vi "Save.vi"(8 "error in (no error)":errorcluster, 9 "new command":string, 10 "Msg in":T1, 11 "FakePressureController in":refnum<class "SMC100.lvclass">) -> (0 "error out":errorcluster, 1 "Path":path, 2 "Msg out":T1, 3 "FakePressureController out":refnum<class "SMC100.lvclass">, 4 "new command":string)   [LabVIEW 2020, in "SMC100.lvclass"]
uses:
  SMC100.lvclass
  DriverMsg.ctl
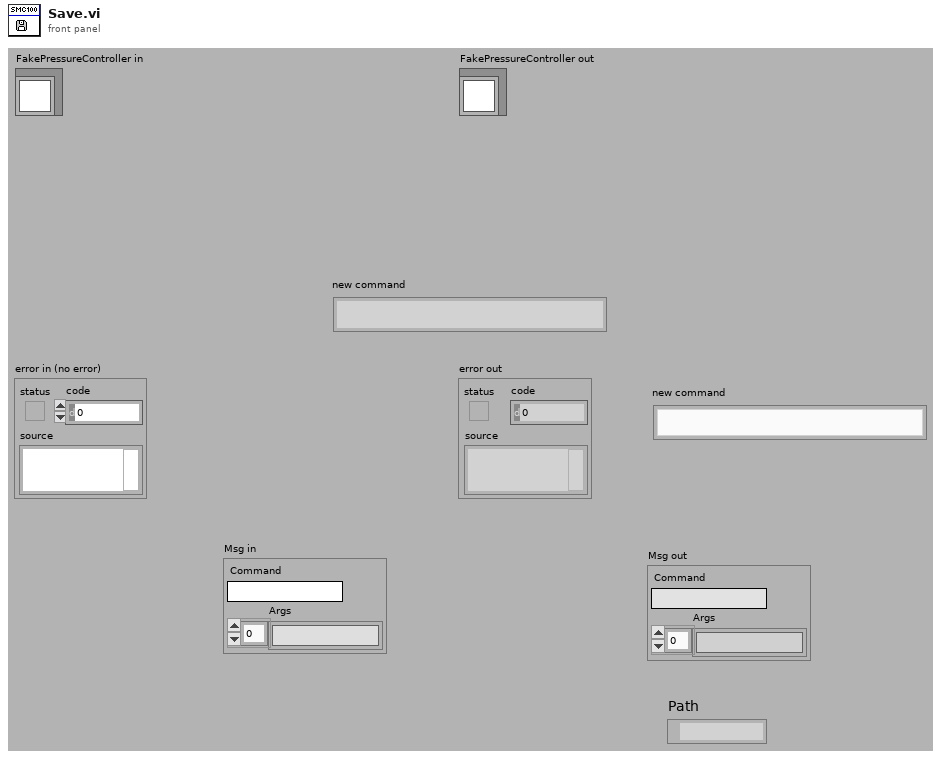
[diagram p1: front panel]
types:
  T1 = typedef "DriverMsg.ctl" = cluster{"Command":string, "Args":string[]}
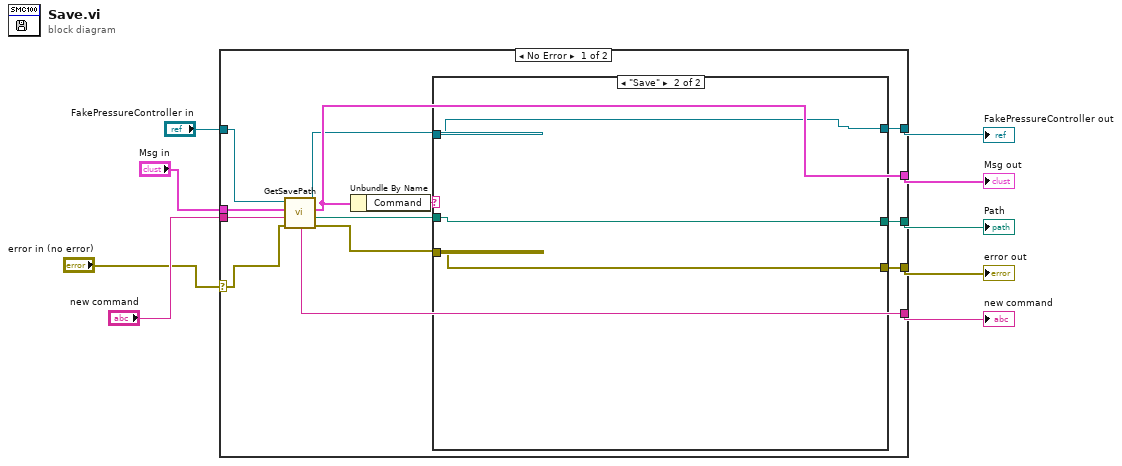
[diagram p0: block diagram]
diagram:
  n1 = case shown="No Error" "error in (no error)" {
    selector: "error in (no error)" -> [w18 w32]
    tunnel: "Msg in" -> [w22 w30]
    tunnel: "new command" -> [w21 w31]
    tunnel: [w20 w31] -> w7
    tunnel: [w12 w32] -> w6
    tunnel: [w10 _] -> w5
    tunnel: [w17 w30] -> w4
    tunnel: "FakePressureController in" -> [w19 w29]
    tunnel: [w14 w29] -> w2
    frame No Error {
      n2 = call-dynamic "GetSavePath.vi"("error in (no error)"=w18, "new command"=w21, "Msg in"=w22, "BaseDriver in"=w19) -> ("error out"=w13:errorcluster, "Path"=w11:path, "Msg out"=w17:T1, "BaseDriver out"=w15:refnum<class "SMC100.lvclass">, "new command"=w20:string)  [unwired: 3 in]
      n3 = Unbundle By Name(w17) -> ("Command"=w16:string)
      n4 = case shown="\"Save\"" w16 {
        tunnel: w15 -> [w25 w28]
        tunnel: [w25 w28] -> w14
        tunnel: w13 -> [w24 w27]
        tunnel: [w24 w27] -> w12
        tunnel: w11 -> [w23 w26]
        tunnel: [w23 w26] -> w10
        frame "False", Default {
        }
        frame "Save" {
        }
      }
    }
    frame Error {
    }
  }
  "error out" <- w6
  "FakePressureController out" <- w2
  "Path" <- w5
  "Msg out" <- w4
  "new command" <- w7
